vi "LabviewMonitoringApplication.vi"() -> ()   [LabVIEW 2024]
uses:
  <vilib>/Utility/error.llb/Trim Whitespace One-Sided.vi
  <vilib>/Instr/_visa.llb/VISA Configure Serial Port (Instr).vi
panel:
  out "CONTROL PANEL":enum32{"DASHBOARD", "SERIAL PORT  Settings"}(tab)
  out "Snapshot data":string
  out "Waveform Chart":T1(graph)
  out "return count read":u32
  in  "STOP":bool=TRUE
  in  "milliseconds to wait":u32=1000
  out "VISA resource name out read":refnum<visa-resource-name>="COM32"
  in  "Start Measurement":bool=TRUE
  out "READ BUFFER":string
  out "Prog. Cnt":i64
  out "AdcValue":dbl
  out "R0 value (kOHm)":dbl(slide) scale=0.0..10.0 scale format="%.2f"
  out "Volatge":dbl(knob) scale=0.0..3.3
  out "Temperature °C":dbl(slide) scale=0.0..100.0 scale format="%#.2g"
  out "Humidity %":dbl(knob) scale=0.1..100.0 scale format="%#.2g"
  out "Heat Index":dbl(slide) scale=0.0..100.0
  out "iPPM_Smoke":i64(slide) scale=0.0..500.0
  out "iPPM_LPG":i64(slide) scale=0.0..100.0
  out "iPPM_CO":i64(slide) scale=0.0..400.0
  in  "Live Data / Historical Data":bool=TRUE
  in  "Temperature":bool=TRUE
  in  "Humidity":bool=TRUE
  in  "PMM_CO":bool=TRUE
  in  "HeatIndex":bool=TRUE
  in  "PMM_LPG":bool=TRUE
  in  "PMM_Smoke":bool=TRUE
  in  "Save file":bool
  in  "Refresh snapshot data":bool
  in  "file path (use dialog)":path
  out "error out read  from VISA":errorcluster={"status"=TRUE, "code"=-1073807339, "source"="VISA Read in LabviewMonitoringApplication.vi"}
  in  "VISA resource name":refnum<visa-resource-name>="COM32"
  in  "Enable Termination\nChar (T)":bool=TRUE
  in  "timeout (ms)":u32=10000
  in  "baud rate (115200)":u32=115200
  in  "byte count":u32=100
  in  "parity (0:none)":enum16{"None", "Odd", "Even", "Mark", "Space"}(ring)
  in  "data bits (8)":u16=8 min=5 max=8 step=1
  in  "termination char\n(0xA = '\\n' = LF)":u8=10 format="%.0x"
  in  "flow control (0:none)":u16(ring) items=["None", "XON/XOFF", "RTS/CTS", "XON/XOFF & RTS/CTS", "DTR/DSR", "XON/XOFF & DTR/DSR"]
  in  "stop bits (10: 1 bit)":u16(ring)=10 items=["1.0"=10, "1.5"=15, "2.0"=20]
  out "error writing file":errorcluster
  # "Select signals (for live data)"
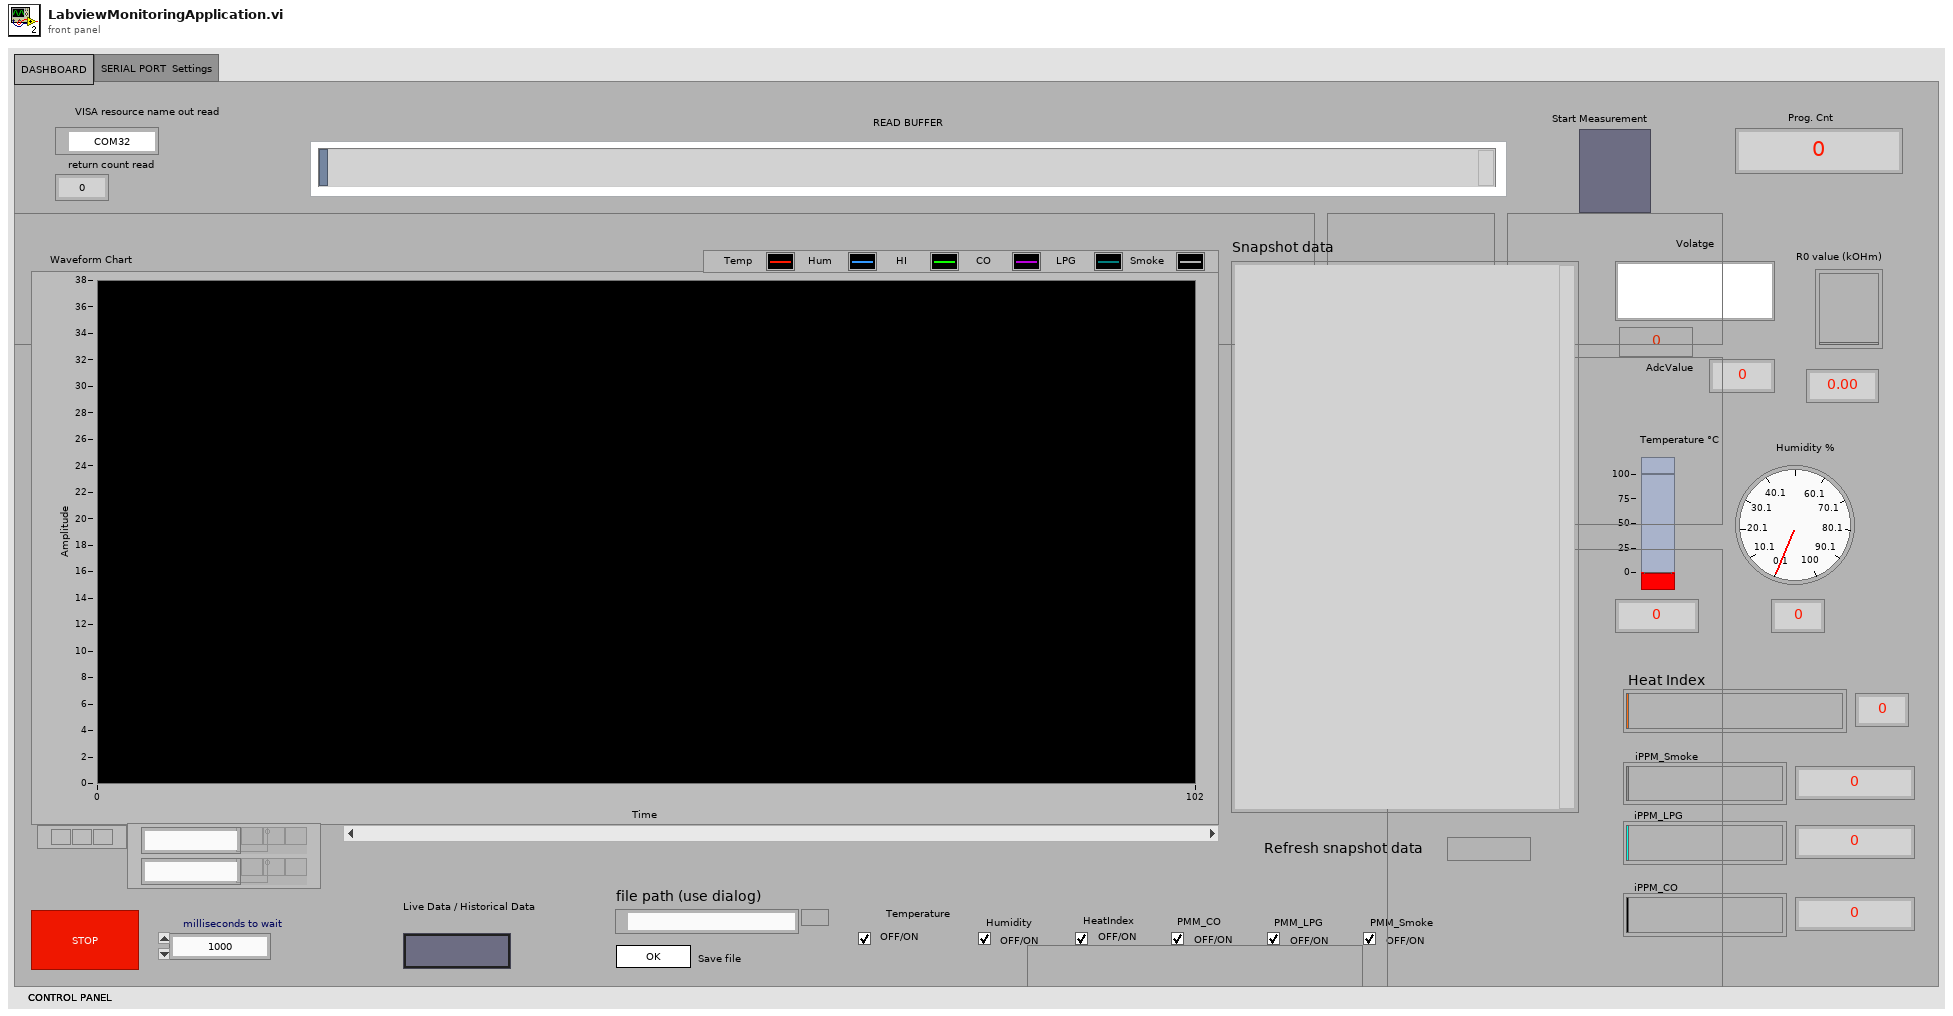
[diagram p1: front panel]
types:
  T1 = cluster{"Temperature °C ":dbl, dbl, dbl, dbl, dbl, dbl}
  T2 = enum16{"open", "replace", "create", "open or create", "replace or create", "replace or create with confirmation"}
  T3 = cluster{"Temperature °C ":dbl, "Humidity %":dbl, "Heat Index":dbl, "iPPM_CO":dbl, "iPPM_LPG":dbl, "iPPM_Smoke":dbl}
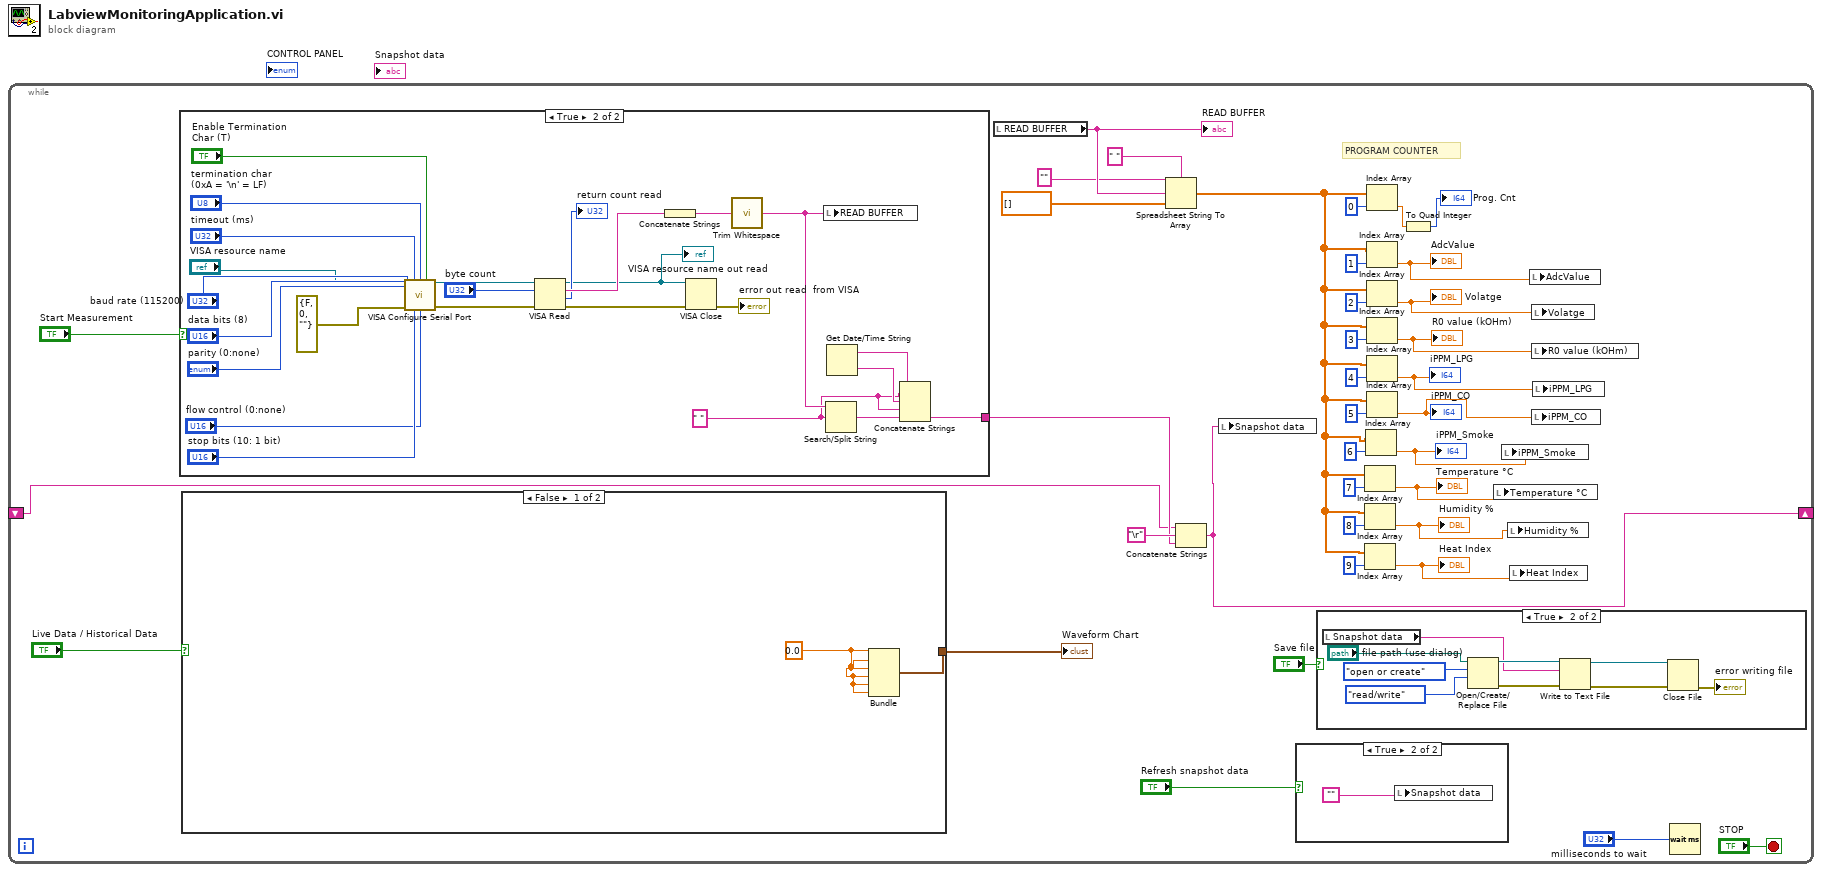
[diagram p0: block diagram]
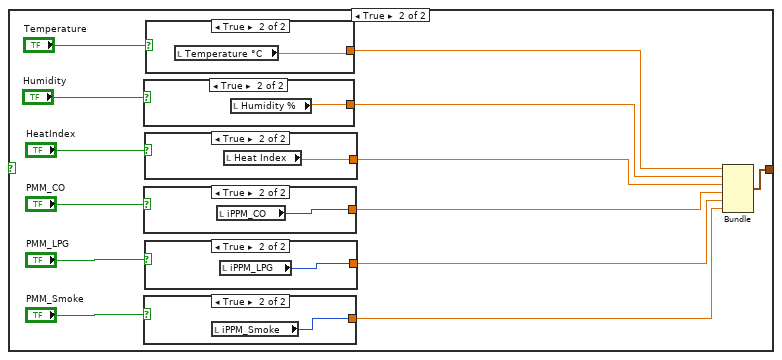
[diagram p4: hidden frame]
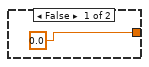
[diagram p5: hidden frame]
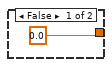
[diagram p6: hidden frame]
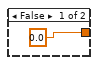
[diagram p7: hidden frame]
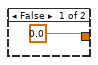
[diagram p8: hidden frame]
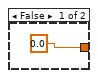
[diagram p9: hidden frame]
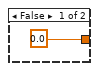
[diagram p10: hidden frame]
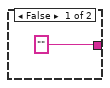
[diagram p11: hidden frame]
diagram:
  n1 = while {
    shift-right: [w2] -> _
    shift-left: _ -> [w3]
    stop <- "STOP" stop-if-true
    # "PROGRAM COUNTER"
    n2 = case shown="True" "Start Measurement" {
      tunnel: ["" w79] -> w4
      frame False {
      }
      frame True {
        w77 = " "
        n3 = call-poly "VISA Configure Serial Port"("VISA resource name"="VISA resource name", "timeout (10sec)"="timeout (ms)", "termination char\n(0xA = '\\n' = LF)"="termination char\n(0xA = '\\n' = LF)", "Enable Termination\nChar (T)"="Enable Termination\nChar (T)", "baud rate (9600)"="baud rate (115200)", "data bits (8)"="data bits (8)", "parity (0:none)"="parity (0:none)", "error in (no error)"=errorcluster {"status"=FALSE, "code"=0, "source"=""}, "stop bits (10: 1 bit)"="stop bits (10: 1 bit)", "flow control (0:none)"="flow control (0:none)") -> ("VISA resource name out"=w93:refnum<visa-resource-name>, "error out"=w92:errorcluster)  [unwired: 4 in]
        n4 = VISA Read(VISA resource name=w93, byte count="byte count", error in (no error)=w92) -> (VISA resource name out=w82:refnum<visa-resource-name>, read buffer=w91:string, return count=→"return count read":u32, error out=w83:errorcluster)
        "VISA resource name out read" <- w82
        n5 = Concatenate Strings(w91) -> (w88:string)
        n6 = VISA Close(VISA resource name=w82, error in (no error)=w83) -> (error out=→"error out read  from VISA":errorcluster)
        n7 = call <vilib>:"Trim Whitespace.vi"("string"=w88) -> ("trimmed string"=w80:string)  [unwired: 1 in]
        n8 = local write "READ BUFFER"(w80) -> ()
        n9 = Search/Split String(string=w80, search string/char (-)=w77) -> (match + rest of string=w81:string)  [unwired: 1 in, 2 out]
        n10 = Get Date/Time String() -> (date string=w76:string, time string=w78:string)  [unwired: 3 in]
        n11 = Concatenate Strings(w76, w77, w78, w77, w81) -> (w79:string)
      }
    }
    n12 = case shown="False" "Live Data / Historical Data" {
      tunnel: [w49 w61] -> w8
      frame False {
        w48 = 0.0
        n13 = Bundle(w48, w48, w48, w48, w48, w48) -> (w49:cluster{dbl, dbl, dbl, dbl, dbl, dbl})  [unwired: 1 in]
      }
      frame True {
        n14 = case shown="True" "Humidity" {
          tunnel: [0.0 w72] -> w54
          frame False {
          }
          frame True {
            n15 = local read "Humidity %"() -> (w72:dbl)
          }
        }
        n16 = case shown="True" "PMM_CO" {
          tunnel: [0.0 w68] -> w52
          frame False {
          }
          frame True {
            n17 = local read "iPPM_CO"() -> (w68:i64)
          }
        }
        n18 = case shown="True" "PMM_Smoke" {
          tunnel: [0.0 w64] -> w50
          frame False {
          }
          frame True {
            n19 = local read "iPPM_Smoke"() -> (w64:i64)
          }
        }
        n20 = case shown="True" "HeatIndex" {
          tunnel: [0.0 w70] -> w53
          frame False {
          }
          frame True {
            n21 = local read "Heat Index"() -> (w70:dbl)
          }
        }
        n22 = case shown="True" "PMM_LPG" {
          tunnel: [0.0 w66] -> w51
          frame False {
          }
          frame True {
            n23 = local read "iPPM_LPG"() -> (w66:i64)
          }
        }
        n24 = case shown="True" "Temperature" {
          tunnel: [0.0 w74] -> w60
          frame False {
          }
          frame True {
            n25 = local read "Temperature °C"() -> (w74:dbl)
          }
        }
        n26 = Bundle("Temperature °C"=w60, "Humidity %"=w54, "Heat Index"=w53, "iPPM_CO"=w52, "iPPM_LPG"=w51, "iPPM_Smoke"=w50) -> (w61:T3)  [unwired: 1 in]
      }
    }
    "Waveform Chart" <- w8
    n27 = local read "READ BUFFER"() -> (w33:string)
    "READ BUFFER" <- w33
    n28 = Spreadsheet String To Array(delimiter (Tab)=" ", format string="", spreadsheet string=w33, array type (2D Dbl)=dbl[] []) -> (array=w19:dbl[])
    n29 = Concatenate Strings(w3, "\r", w4) -> (w2:string)
    n30 = local write "Snapshot data"(w2) -> ()
    n31 = case shown="True" "Refresh snapshot data" {
      frame False {
      }
      frame True {
        n32 = local write "Snapshot data"("") -> ()
      }
    }
    n33 = case shown="True" "Save file" {
      frame False {
      }
      frame True {
        n34 = local read "Snapshot data"() -> (w41:string)
        n35 = Open/Create/Replace File(file path (use dialog)="file path (use dialog)", operation (0:open)=T2."open or create", access (0:read/write)=enum16{"read/write", "read-only", "write-only"}."read/write") -> (refnum out=w46:refnum<file>, error out=w45:errorcluster)  [unwired: 3 in, 1 out]
        n36 = Write to Text File(file (use dialog)=w46, text=w41, error in=w45) -> (refnum out=w43:refnum<file>, error out=w44:errorcluster)  [unwired: 1 in, 1 out]
        n37 = Close File(refnum=w43, error in=w44) -> (error out=→"error writing file":errorcluster)  [unwired: 1 out]
      }
    }
    n38 = Index Array(array=w19, index=7) -> (element=w11:dbl)
    "Temperature °C" <- w11
    n39 = Index Array(array=w19, index=8) -> (element=w12:dbl)
    "Humidity %" <- w12
    n40 = Index Array(array=w19, index=9) -> (element=w13:dbl)
    "Heat Index" <- w13
    n41 = Index Array(array=w19, index=6) -> (element=w10:dbl)
    "iPPM_Smoke" <- w10
    n42 = Index Array(array=w19, index=0) -> (element=w30:dbl)
    n43 = Index Array(array=w19, index=1) -> (element=w18:dbl)
    "AdcValue" <- w18
    n44 = Index Array(array=w19, index=2) -> (element=w17:dbl)
    "Volatge" <- w17
    n45 = Index Array(array=w19, index=3) -> (element=w16:dbl)
    "R0 value (kOHm)" <- w16
    n46 = Index Array(array=w19, index=4) -> (element=w15:dbl)
    "iPPM_LPG" <- w15
    n47 = Index Array(array=w19, index=5) -> (element=w14:dbl)
    "iPPM_CO" <- w14
    n48 = To Quad Integer(1:w30) -> (0:→"Prog. Cnt":i64)
    n49 = local write "Temperature °C"(w11) -> ()
    n50 = local write "iPPM_Smoke"(w10) -> ()
    n51 = local write "Humidity %"(w12) -> ()
    n52 = local write "Heat Index"(w13) -> ()
    n53 = local write "AdcValue"(w18) -> ()
    n54 = local write "Volatge"(w17) -> ()
    n55 = local write "R0 value (kOHm)"(w16) -> ()
    n56 = local write "iPPM_CO"(w14) -> ()
    n57 = local write "iPPM_LPG"(w15) -> ()
    n58 = Wait (ms)(milliseconds to wait="milliseconds to wait") -> ()  [unwired: 1 out]
  }
